vi "Overflow-Safe Millis Elapsed.vi"(1 "now":u32, 2 "previous":u32) -> (6 "elapsed":u32)   [LabVIEW 2020]
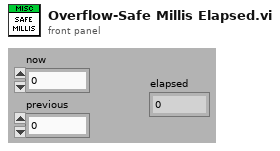
[diagram p1: front panel]
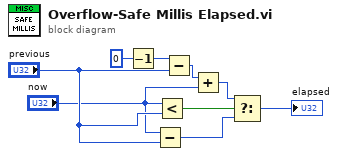
[diagram p0: block diagram]
diagram:
  n1 = Decrement(x=u32 0 ("millisecond timer value")) -> (x-1=w3:u32)
  n2 = Subtract(x="now", y="previous") -> (x-y=w8:u32)
  n3 = Less?(x="now", y="previous") -> (x < y?=w2:bool)
  n4 = Subtract(x=w3, y="previous") -> (x-y=w4:u32)
  n5 = Add(x=w4, y="now") -> (x+y=w5:u32)
  n6 = Select(t=w5, s=w2, f=w8) -> (s? t:f=→"elapsed":u32)
